vi "Get Target String.vi"(8 "error in (no error)":errorcluster, 11 "Search Result in":refnum<class "Search Result.lvclass">) -> (0 "error out":errorcluster, 2 "Target":string, 3 "Search Result out":refnum<class "Search Result.lvclass">)   [LabVIEW 2020, in "Better Search.lvlib" / "Search Result.lvclass"]
uses:
  Search Result.lvclass
  Search Result.lvclass/Search Result.ctl
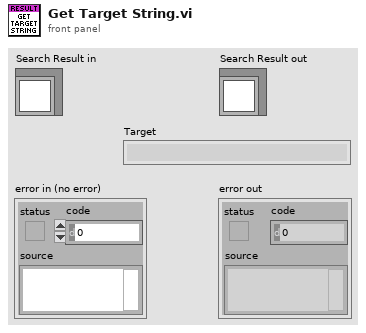
[diagram p1: front panel]
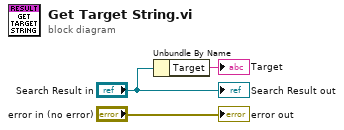
[diagram p0: block diagram]
diagram:
  n1 = Unbundle By Name("Search Result in") -> ("Target"=→"Target":string)
  "error out" <- "error in (no error)"
  "Search Result out" <- "Search Result in"
